vi "Test Control Experiment.vi"() -> ()   [LabVIEW 2019, in "Control Experiment.lvclass"]
uses:
  Control Experiment/Control Experiment.lvclass
  <userlib>/LevyLab/Instrument Framework/Instrument Types/Cryostat/Instrument.Cryostat.lvclass
panel:
  in  "stop":bool
  out "B Field (T)":dbl
  out "Temperature (K)":dbl
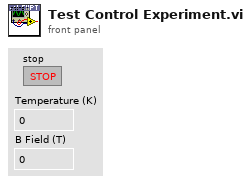
[diagram p1: front panel]
types:
  T1 = typedef "Control Experiment.lvclass/Instrument Classes--cluster.ctl" = cluster{"KH7008":refnum<class "Instrument.KH7008.lvclass">[], "Lockin":refnum<class "Instrument.Lockin.lvclass">, "Temperature":refnum<class "Instrument.Cryostat.lvclass">, "Magnet":refnum<class "Instrument.Cryostat.lvclass">, "Rotator":refnum<class "Instrument.Cryostat.lvclass">, "Level":refnum<class "Instrument.Cryostat.lvclass">, "Capacitance Bridge":refnum<class "Instrument.CBridge.lvclass">, "Delay Line":refnum<class "Instrument.DelayLine.lvclass">, "Strain Cell":refnum<class "Instrument.Strain.lvclass">, "VNA":refnum<class "Instrument.VNA.lvclass">, "Voltage Source":refnum<class "Instrument.VSource.lvclass">}
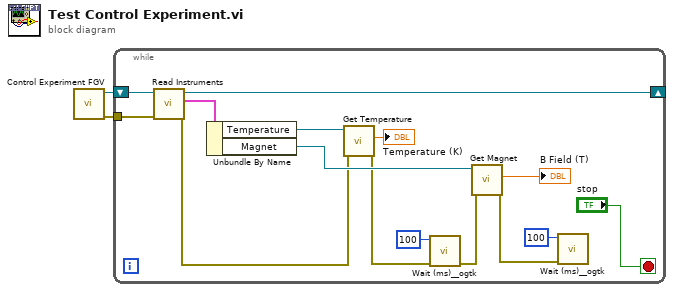
[diagram p0: block diagram]
diagram:
  n1 = call "Control Experiment FGV.vi"() -> ("error out"=w1:errorcluster, "Control Experiment.lvclass out"=w2:refnum<class "Control Experiment.lvclass">)  [unwired: 10 in]
  n2 = while {
    tunnel: w1 -> [w16]
    shift-right: [w6] -> _
    shift-left: w2 -> [w17]
    stop <- "stop" stop-if-true
    n3 = call "Read Instruments.vi"("error in (no error)"=w16, "Control Experiment in"=w17) -> ("error out"=w5:errorcluster, "Instruments"=w15:T1, "Control Experiment out"=w6:refnum<class "Control Experiment.lvclass">)  [unwired: 7 in]
    n4 = Unbundle By Name(w15) -> ("Temperature"=w14:refnum<class "Instrument.Cryostat.lvclass">, "Magnet"=w13:refnum<class "Instrument.Cryostat.lvclass">)
    n5 = call-dynamic "Get Temperature.vi"("error in (no error)"=w5, "Instrument.Cryostat in"=w14) -> ("error out"=w4:errorcluster, "Temperature (K)"=→"Temperature (K)":dbl)  [unwired: 5 in, 3 out]
    n6 = call <userlib>:"Wait (ms)__ogtk.vi"("error in (no error)"=w4, "milliseconds to wait"=u32 100) -> ("error out"=w10:errorcluster)  [unwired: 8 in, 1 out]
    n7 = call-dynamic "Get Magnet.vi"("error in (no error)"=w10, "Instrument.Cryostat in"=w13) -> ("error out"=w7:errorcluster, "B Field (T)"=→"B Field (T)":dbl)  [unwired: 5 in, 3 out]
    n8 = call <userlib>:"Wait (ms)__ogtk.vi"("error in (no error)"=w7, "milliseconds to wait"=u32 100) -> ()  [unwired: 8 in, 2 out]
  }
